vi "VIve LabVIEW_Text if empty.vi"(2 "Text in":string, 6 "Text if empty":string="Not Used") -> (12 "Property.Disabled":T1(ring)=enum."Disabled & Grayed", 16 "Text out":string="Not used")   [LabVIEW 2009]
doc: "This VI outputs text depending of the Text input\n\nIf Text input is >0 (Space bars, Tabs, etc are trimmed in both sides), then the output text will be equal as the text input.\n\nIf the text input is <=0 The text output will be equal as the : Text If empty control value\n\n\nText If empty default value is : Not Used\n\n\n<b> VIve LabVIEW </b>"
panel:
  # "Outputs"
  # "Inputs"
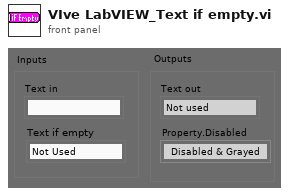
[diagram p1: front panel]
types:
  T1 = enum16{"Enable", "Disabled", "Disabled & Grayed"}
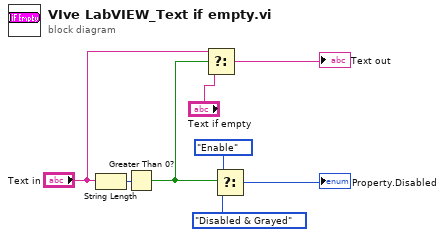
[diagram p0: block diagram]
diagram:
  n1 = String Length(string="Text in") -> (length=w8:i32)
  n2 = Greater Than 0?(x=w8) -> (x > 0?=w4:bool)
  n3 = Select(t="Text in", s=w4, f="Text if empty") -> (s? t:f=→"Text out":string)
  n4 = Select(t=T1."Enable", s=w4, f=T1."Disabled & Grayed") -> (s? t:f=→"Property.Disabled":T1)
